vi "bin calibrtion.vi"(8 "error in":errorcluster, 10 "Param Calibrazione":T1, 11 "Sum Spectrum":cluster{"Ramp Pattern":dbl[], "Array":i32[]}[](graph)) -> (0 "error out":errorcluster, 3 "Sum Spectrum Out":cluster{"Ramp Pattern":dbl[], "Array":i32[]}[](graph))   [LabVIEW 2023]
uses:
  control/param_calibrazione.ctl
  <vilib>/Analysis/1siggen.llb/Ramp Pattern by Samples.vi
  <vilib>/Analysis/NI_AALBase.lvlib
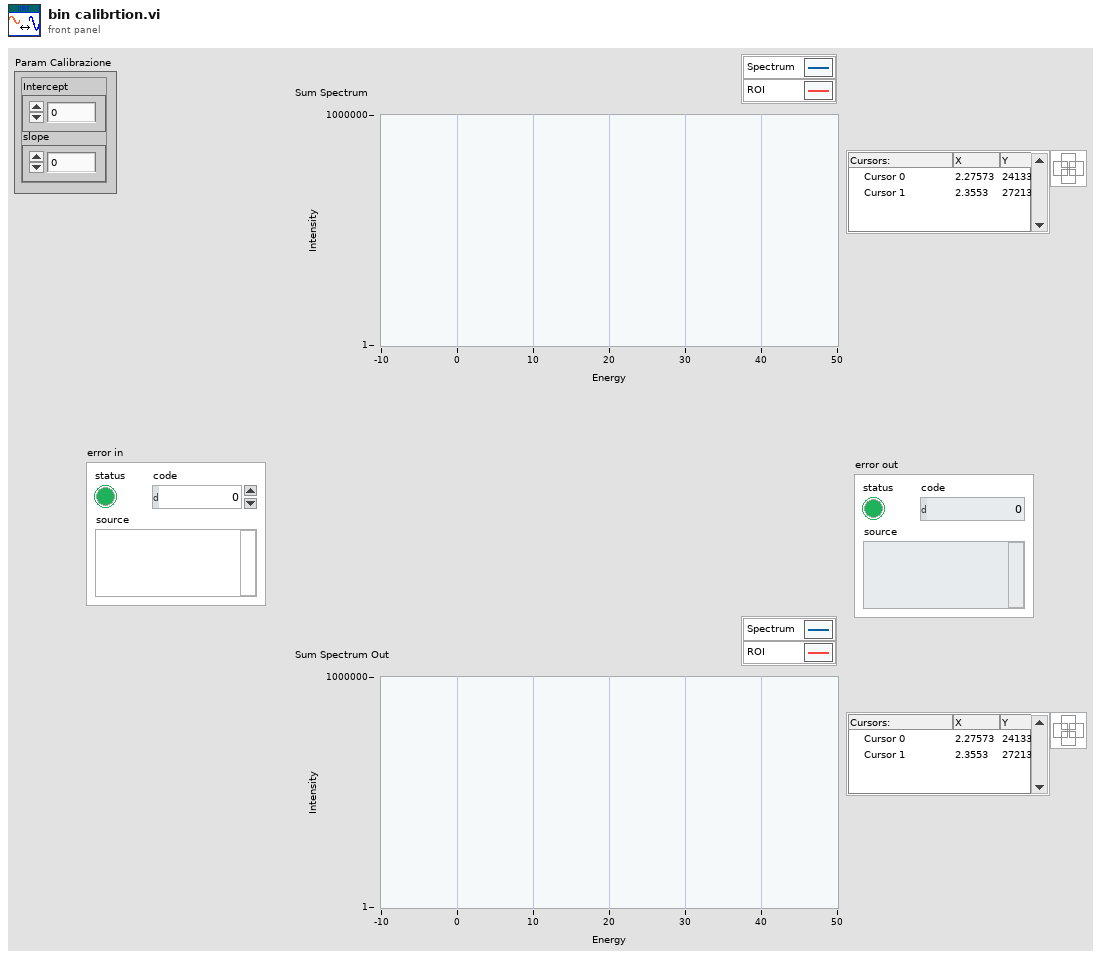
[diagram p1: front panel]
types:
  T1 = typedef "param_calibrazione.ctl" = cluster{"Intercept":dbl, "slope":dbl}
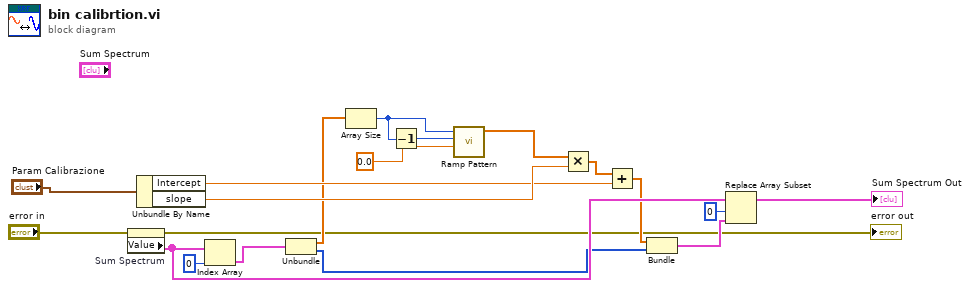
[diagram p0: block diagram]
diagram:
  n1 = property on="Sum Spectrum" class="XYGraph (strict)"(error in="error in") -> (error out=→"error out":errorcluster, "Value"=w17:cluster{"Ramp Pattern":dbl[], "Array":i32[]}[])  [unwired: 1 in, 1 out]
  n2 = Unbundle By Name("Param Calibrazione") -> ("Intercept"=w13:dbl, "slope"=w14:dbl)
  n3 = Index Array(array=w17, index=0) -> (element=w16:cluster{"Ramp Pattern":dbl[], "Array":i32[]})
  n4 = Unbundle(w16) -> ("Ramp Pattern"=w9:dbl[], "Array"=w10:i32[])
  n5 = Array Size(array=w9) -> (size(s)=w8:i32)
  n6 = Decrement(x=w8) -> (x-1=w7:i32)
  n7 = call-poly <vilib>:"Ramp Pattern.vi"("start"=0.0, "end"=w7, "samples"=w8) -> ("Ramp Pattern"=w12:dbl[])  [unwired: 7 in, 1 out]
  n8 = Multiply(x=w12, y=w14) -> (x*y=w5:dbl[])
  n9 = Add(x=w5, y=w13) -> (x+y=w11:dbl[])
  n10 = Bundle(w11, "Array"=w10) -> (w19:cluster{dbl[], "Array":i32[]})  [unwired: 1 in]
  n11 = Replace Array Subset(array=w17, new element=w19, index=0) -> (→"Sum Spectrum Out":cluster{"Ramp Pattern":dbl[], "Array":i32[]}[])
